vi "DAQNavi Read (Analog 1D U16 NChan NSamp).vi"(8 "error in (no error)":errorcluster, 9 "number of samples per channel to read":u32=1000, 10 "timeout":dbl=10.0 format="%0.2f", 11 "task in":i32) -> (0 "error out":errorcluster, 1 "markBuf":cluster{"DataIndex":i64, "SrcId":i64}[](array[cluster]), 2 "data":u16[](array[numeric]), 3 "task out":i32)   [LabVIEW 2020]
uses:
  DAQNavi_LV.dll
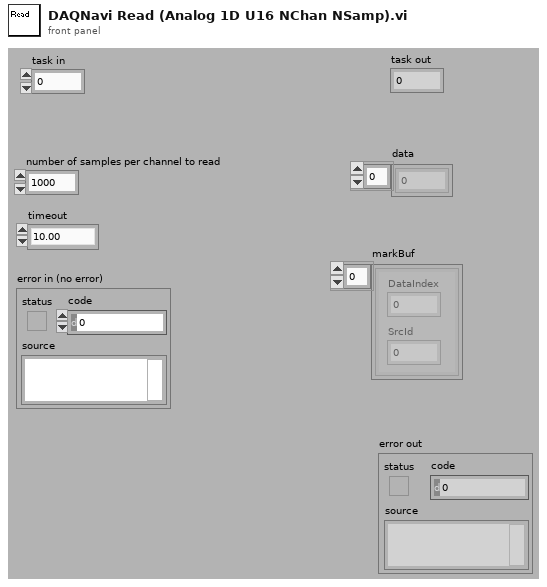
[diagram p1: front panel]
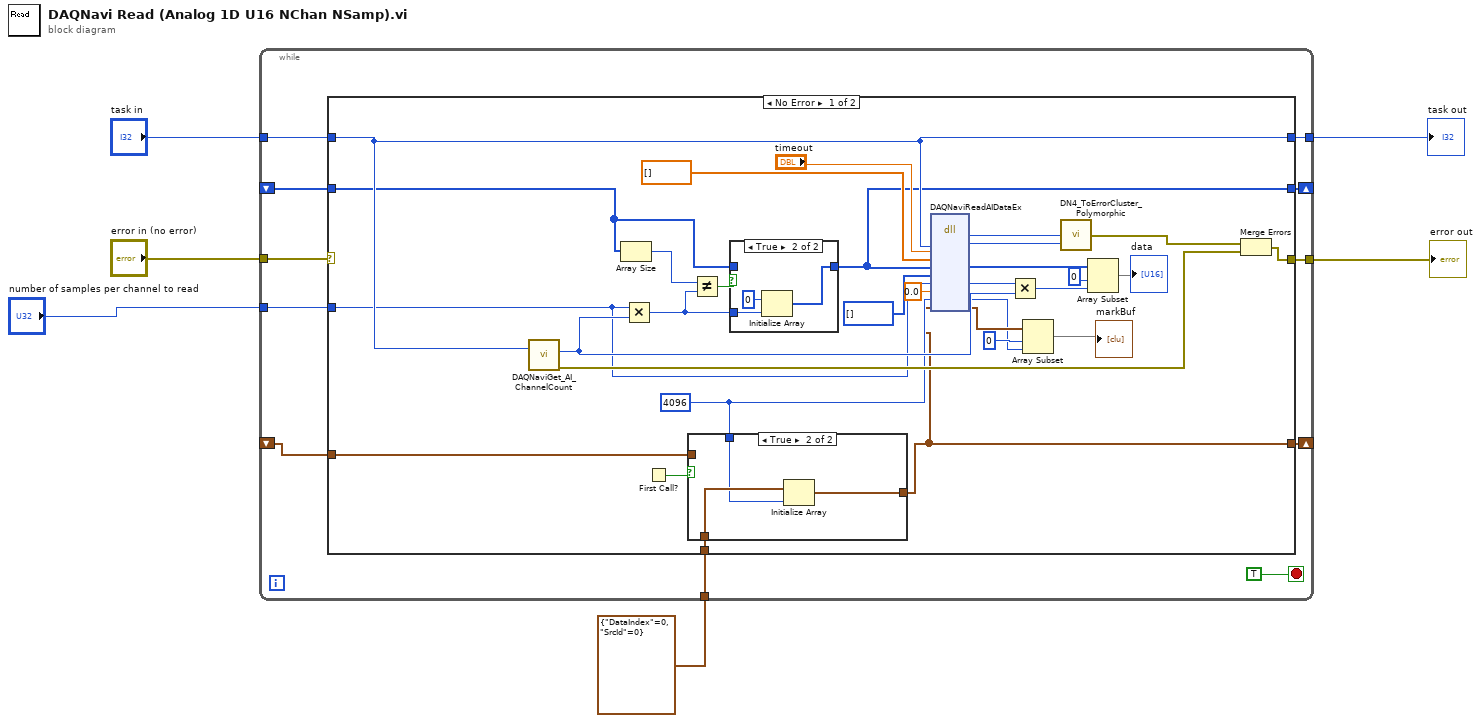
[diagram p0: block diagram]
diagram:
  n1 = while {
    tunnel: "task in" -> [w17]
    tunnel: "error in (no error)" -> [w16]
    tunnel: [w15] -> w4
    tunnel: [w14] -> w3
    tunnel: "number of samples per channel to read" -> [w13]
    shift-right: [w11] -> _
    shift-left: _ -> [w10]
    shift-right: [w8] -> _
    shift-left: _ -> [w7]
    tunnel: cluster{"DataIndex":i64, "SrcId":i64} {"DataIndex"=0, "SrcId"=0} -> [w9]
    stop <- TRUE stop-if-true
    n2 = case shown="No Error" w16 {
      selector: w16 -> [_ w59]
      tunnel: w17 -> [w40 w60]
      tunnel: [w40 w60] -> w15
      tunnel: [w37 w59] -> w14
      tunnel: w13 -> [w32 _]
      tunnel: [w29 w58] -> w11
      tunnel: w10 -> [w28 w58]
      tunnel: w9 -> [w25 _]
      tunnel: [w22 w57] -> w8
      tunnel: w7 -> [w23 w57]
      frame No Error {
        w24 = 4096 ("element")
        n3 = call "DAQNaviGet_AI_ChannelCount.vi"("task in"=w40) -> ("error out"=w38:errorcluster, "channel count"=w35:i32)  [unwired: 1 in, 8 out]
        n4 = Array Size(array=w28) -> (size(s)=w31:i32)
        n5 = Multiply(x=w32, y=w35) -> (x*y=w41:u32)
        n6 = First Call?() -> (First Call?: T/F=w26:bool)
        n7 = case shown="True" w26 {
          tunnel: w25 -> [_ w52]
          tunnel: w24 -> [_ w51]
          tunnel: [w49 w50] -> w22
          tunnel: w23 -> [w49 _]
          frame False {
          }
          frame True {
            n8 = Initialize Array(w52, w51) -> (w50:cluster{"DataIndex":i64, "SrcId":i64}[])
          }
        }
        n9 = Not Equal?(x=w31, y=w41) -> (x != y?=w30:bool)
        n10 = case shown="True" w30 {
          tunnel: w41 -> [_ w55]
          tunnel: [w53 w54] -> w29
          tunnel: w28 -> [w53 _]
          frame False {
          }
          frame True {
            n11 = Initialize Array(u16 0 ("element"), w55) -> (w54:u16[])
          }
        }
        n12 = dll-call lib="DAQNavi_LV.dll" fn="DAQNaviReadAIDataEx"("taskID"=w40, "timeout"="timeout", "scaledData"=dbl[] [], "rawData16"=w29, "rawData32"=u32[] [], "samples"=w32, "startTime"=0.0, "markCount"=w24, "markBuf"=w22) -> ("return type"=w45:i32, "taskID"=w33:i32, "rawData16"=w44:u16[], "samples"=w36:u32, "markCount"=w19:i32, "markBuf"=w21:cluster{"DataIndex":i64, "SrcId":i64}[])  [unwired: 4 in, 5 out]
        n13 = Multiply(x=w36, y=w35) -> (x*y=w34:u32)
        n14 = Array Subset(array=w21, index=0, length=w19) -> (→"markBuf":cluster{"DataIndex":i64, "SrcId":i64}[])
        n15 = call "DN4_ToErrorCluster_Polymorphic.vi"("task id"=w33, "error code"=w45) -> ("error out"=w39:errorcluster)  [unwired: 3 out]
        n16 = Array Subset(array=w44, index=0, length=w34) -> (→"data":u16[])
        n17 = Merge Errors(w39, w38) -> (w37:errorcluster)
      }
      frame Error {
      }
    }
  }
  "task out" <- w4
  "error out" <- w3
